vi "Chebyshev Window (DBL).vi"(10 "lobe ratio (dB)":dbl=60.0, 11 "X":dbl[](array[numeric])) -> (0 "error":i32, 3 "Windowed X":dbl[](array[numeric]))   [LabVIEW 2014, in "NI_AALPro.lvlib"]
doc: "Applies an asymmetrical Dolph-Chebyshev window to the input sequence <B>X</B>. Wire data to the <B>X</B> input to determine the polymorphic instance to use or manually select the instance."
uses:
  NI_AALPro.lvlib
  lvanlys.dll
panel:
  # "Dolph-Chebyshev Window"
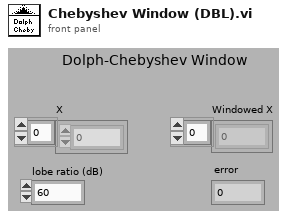
[diagram p1: front panel]
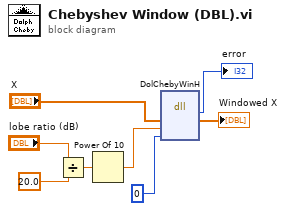
[diagram p0: block diagram]
diagram:
  n1 = Divide(x="lobe ratio (dB)", y=20.0) -> (x/y=w4:dbl)
  n2 = Power Of 10(x=w4) -> (10^x=w2:dbl)
  n3 = dll-call lib="C:/Program Files (x86)/National Instruments/LabVIEW 2014/resource/lvanlys.*" fn="DolChebyWinH"("X"="X", "s"=w2, "sym"=0) -> (→"error":i32, "X"=→"Windowed X":dbl[])  [unwired: 5 in, 2 out]
